vi "Teleop.vi"(10 "Match Info":T1={"Autonomous Elapsed Seconds"=0.0, "TeleOp Elapsed Seconds"=0.0, "Disabled Elapsed Seconds"=0.0, "Visited Autonomous"=FALSE, "Visited TeleOp"=FALSE, "Visited Disabled"=FALSE, "Autonomous Settings"={"Autonomous Style"=enum."Independent", "VI Refnum"=refnum}}, 11 "Call Context":T2) -> ()   [LabVIEW 2013]
doc: "This VI is called for each TeleOp packet received from the DS where the robot is not disabled. It is often used to read from the joysticks and update I/O or to update setpoints for timed control loops. It should complete and return within 20 milliseconds or it may miss DS packets."
uses:
  <vilib>/Rock Robotics/WPI/DriverStation/WPI_DriverStationDerivedRobotMode.ctl
  <vilib>/Rock Robotics/WPI/DriverStation/WPI_DriverStationMatch Info.ctl
  <vilib>/Rock Robotics/WPI/DriverStation/DriverStationLCD/WPI_DriverStationLCDLCDLine.ctl
  Robot Global Data.vi
  <vilib>/Rock Robotics/WPI/Joystick/WPI_JoystickGetSetRefNum.vi
  <vilib>/Rock Robotics/WPI/RobotDrive/WPI_RobotDriveGetSetRefNum.vi
  <vilib>/Rock Robotics/WPI/Solenoid/WPI_SolenoidSetEnum.vi
  <vilib>/Rock Robotics/WPI/Solenoid/WPI_SolenoidValue.ctl
panel:
  out "Numeric 1":dbl(slide) scale=0.0..100.0
  out "Boolean 2":bool
  out "Boolean 1":bool
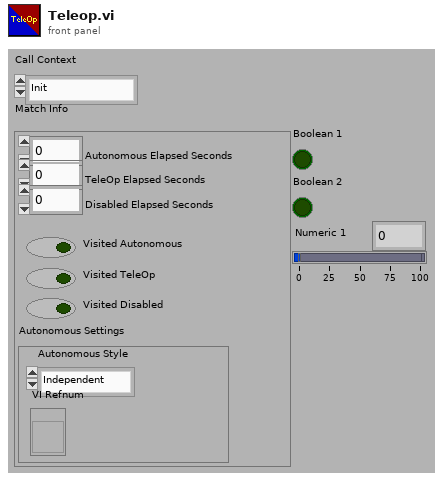
[diagram p1: front panel]
types:
  T1 = typedef "WPI_DriverStationMatch Info.ctl" = cluster{"Autonomous Elapsed Seconds":dbl, "TeleOp Elapsed Seconds":dbl, "Disabled Elapsed Seconds":dbl, "Visited Autonomous":bool, "Visited TeleOp":bool, "Visited Disabled":bool, "Autonomous Settings":cluster{"Autonomous Style":enum16{"Iterative", "Independent"}, "VI Refnum":refnum<vi>}}
  T2 = typedef "WPI_DriverStationDerivedRobotMode.ctl" = enum16{"Init", "Execute", "Stop"}
  T3 = typedef "WPI_DriverStationLCDLCDLine.ctl" = enum16{"Main - Line 1", "User - Line 2", "User - Line 3", "User - Line 4", "User - Line 5", "User - Line 6"}
  T4 = typedef "WPI_JoystickDevRef.ctl" = cluster{"Device":T5}
  T5 = typedef "WPI_JoystickDeviceEnum.ctl" = enum16{"USB 1", "USB 2", "USB 3", "USB 4", "Kinect 1", "Kinect 2"}
  T6 = typedef "WPI_JoystickButtonState.ctl" = cluster{"Button 1":bool, "Button 2":bool, "Button 3":bool, "Button 4":bool, "Button 5":bool, "Button 6":bool, "Button 7":bool, "Button 8":bool, "Button 9":bool, "Button 10":bool, "Button 11":bool, "Button 12":bool}
  T7 = cluster{"axis 1 (x)":dbl, "axis 2 (y)":dbl, "axis 3 (throttle)":dbl, "axis 4":dbl, "axis 5":dbl, "axis 6":dbl}
  T8 = typedef "WPI_SolenoidValue.ctl" = enum16{"Off", "On", "Forward", "Reverse"}
  T9 = typedef "WPI_SolenoidDevRef.ctl" = cluster{"DevStatus":errorcluster, "Solenoid Module":T10, "Forward Solenoid Channel":T11, "Reverse Solenoid Channel":T11}
  T10 = typedef "FPGA_TypedefSolenoidModule.ctl" = enum16{"Solenoid Module 1", "Solenoid Module 2"}
  T11 = typedef "WPI_SolenoidChannel.ctl" = enum8{"Solenoid 1", "Solenoid 2", "Solenoid 3", "Solenoid 4", "Solenoid 5", "Solenoid 6", "Solenoid 7", "Solenoid 8", "Invalid"}
  T12 = typedef "WPI_RobotDriveDevRef.ctl" = cluster{"DevStatus":errorcluster, "Motors[]":T13[], "Square Inputs":bool, "Max Output":dbl, "Isochronous":bool}
  T13 = typedef "WPI_MotorControlDeviceRef.ctl" = cluster{"DeviceStatus":errorcluster, "Type":enum16{"PWM", "CAN"}, "PWM":cluster{"Digital Module":T14, "PWM Channel":T15, "DeadBand":T16}, "CAN":cluster{"Device Number":u8, "Control Mode":T17, "Semaphore":T18, "Max Vout":dbl}, "Invert":bool, "TransformRef":T19, "InvTransformRef":T19}
  T14 = typedef "FPGA_TypedefDigitalModule.ctl" = enum16{"Digital Module 1", "Digital Module 2"}
  T15 = typedef "FPGA_DIOPWMChannel.ctl" = enum8{"PWM 1", "PWM 2", "PWM 3", "PWM 4", "PWM 5", "PWM 6", "PWM 7", "PWM 8", "PWM 9", "PWM 10", "Invalid"}
  T16 = typedef "WPI_PWMDeadband.ctl" = cluster{"Name":string, "maxPositivePwm":i32, "minPositivePwm":i32, "centerPwm":i32, "maxNegativePwm":i32, "minNegativePwm":i32, "angularRange":u16}
  T17 = typedef "WPI_CANJaguar_ControlMode.ctl" = enum8{"Percent VBus", "Current", "Speed", "Position", "Voltage"}
  T18 = typedef "Semaphore RefNum" = refnum<k1>
  T19 = typedef "WPI_PWMTransform_ConPane.ctl" = refnum<vi>
  T20 = enum16{"Reset", "Start", "Reset 2", "Manual", "Get ready to Fire", "Disengage Gearbox", "Ready to Fire", "Firing", "Firing Completed", "Reengage Gearbox"}
  T21 = typedef "WPI_DigitalInputDevRef.ctl" = cluster{"DevStatus":errorcluster, "DIO Channel":T22, "Digital Module":T14}
  T22 = typedef "FPGA_DIOChannel.ctl" = enum8{"DIO 1", "DIO 2", "DIO 3", "DIO 4", "DIO 5", "DIO 6", "DIO 7", "DIO 8", "DIO 9", "DIO 10", "DIO 11", "DIO 12", "DIO 13", "DIO 14", "Invalid"}
  T23 = typedef "WPI_ServoDeviceRef.ctl" = cluster{"DeviceStatus":errorcluster, "Digital Module":T14, "PWM Channel":T15, "DeadBand":T16}
  T24 = typedef "WPI_AnalogChannelDevRef.ctl" = cluster{"DevStatus":errorcluster, "Analog Module":T25, "Analog Channel":T26}
  T25 = typedef "FPGA_TypedefAnalogModule.ctl" = enum16{"Analog Module 1", "Analog Module 2"}
  T26 = typedef "FPGA_AIChannel.ctl" = enum8{"AI 1", "AI 2", "AI 3", "AI 4", "AI 5", "AI 6", "AI 7", "AI 8", "Invalid"}
  T27 = typedef "WPI_RelayDevRef.ctl" = cluster{"DevStatus":errorcluster, "Relay Channel":T28, "Digital Module":T14, "Relay Direction":T29}
  T28 = typedef "FPGA_DIORelayChannel.ctl" = enum8{"Relay 1", "Relay 2", "Relay 3", "Relay 4", "Relay 5", "Relay 6", "Relay 7", "Relay 8", "Invalid"}
  T29 = typedef "WPI_RelayDirection.ctl" = enum16{"Both directions", "Forward only", "Reverse only"}
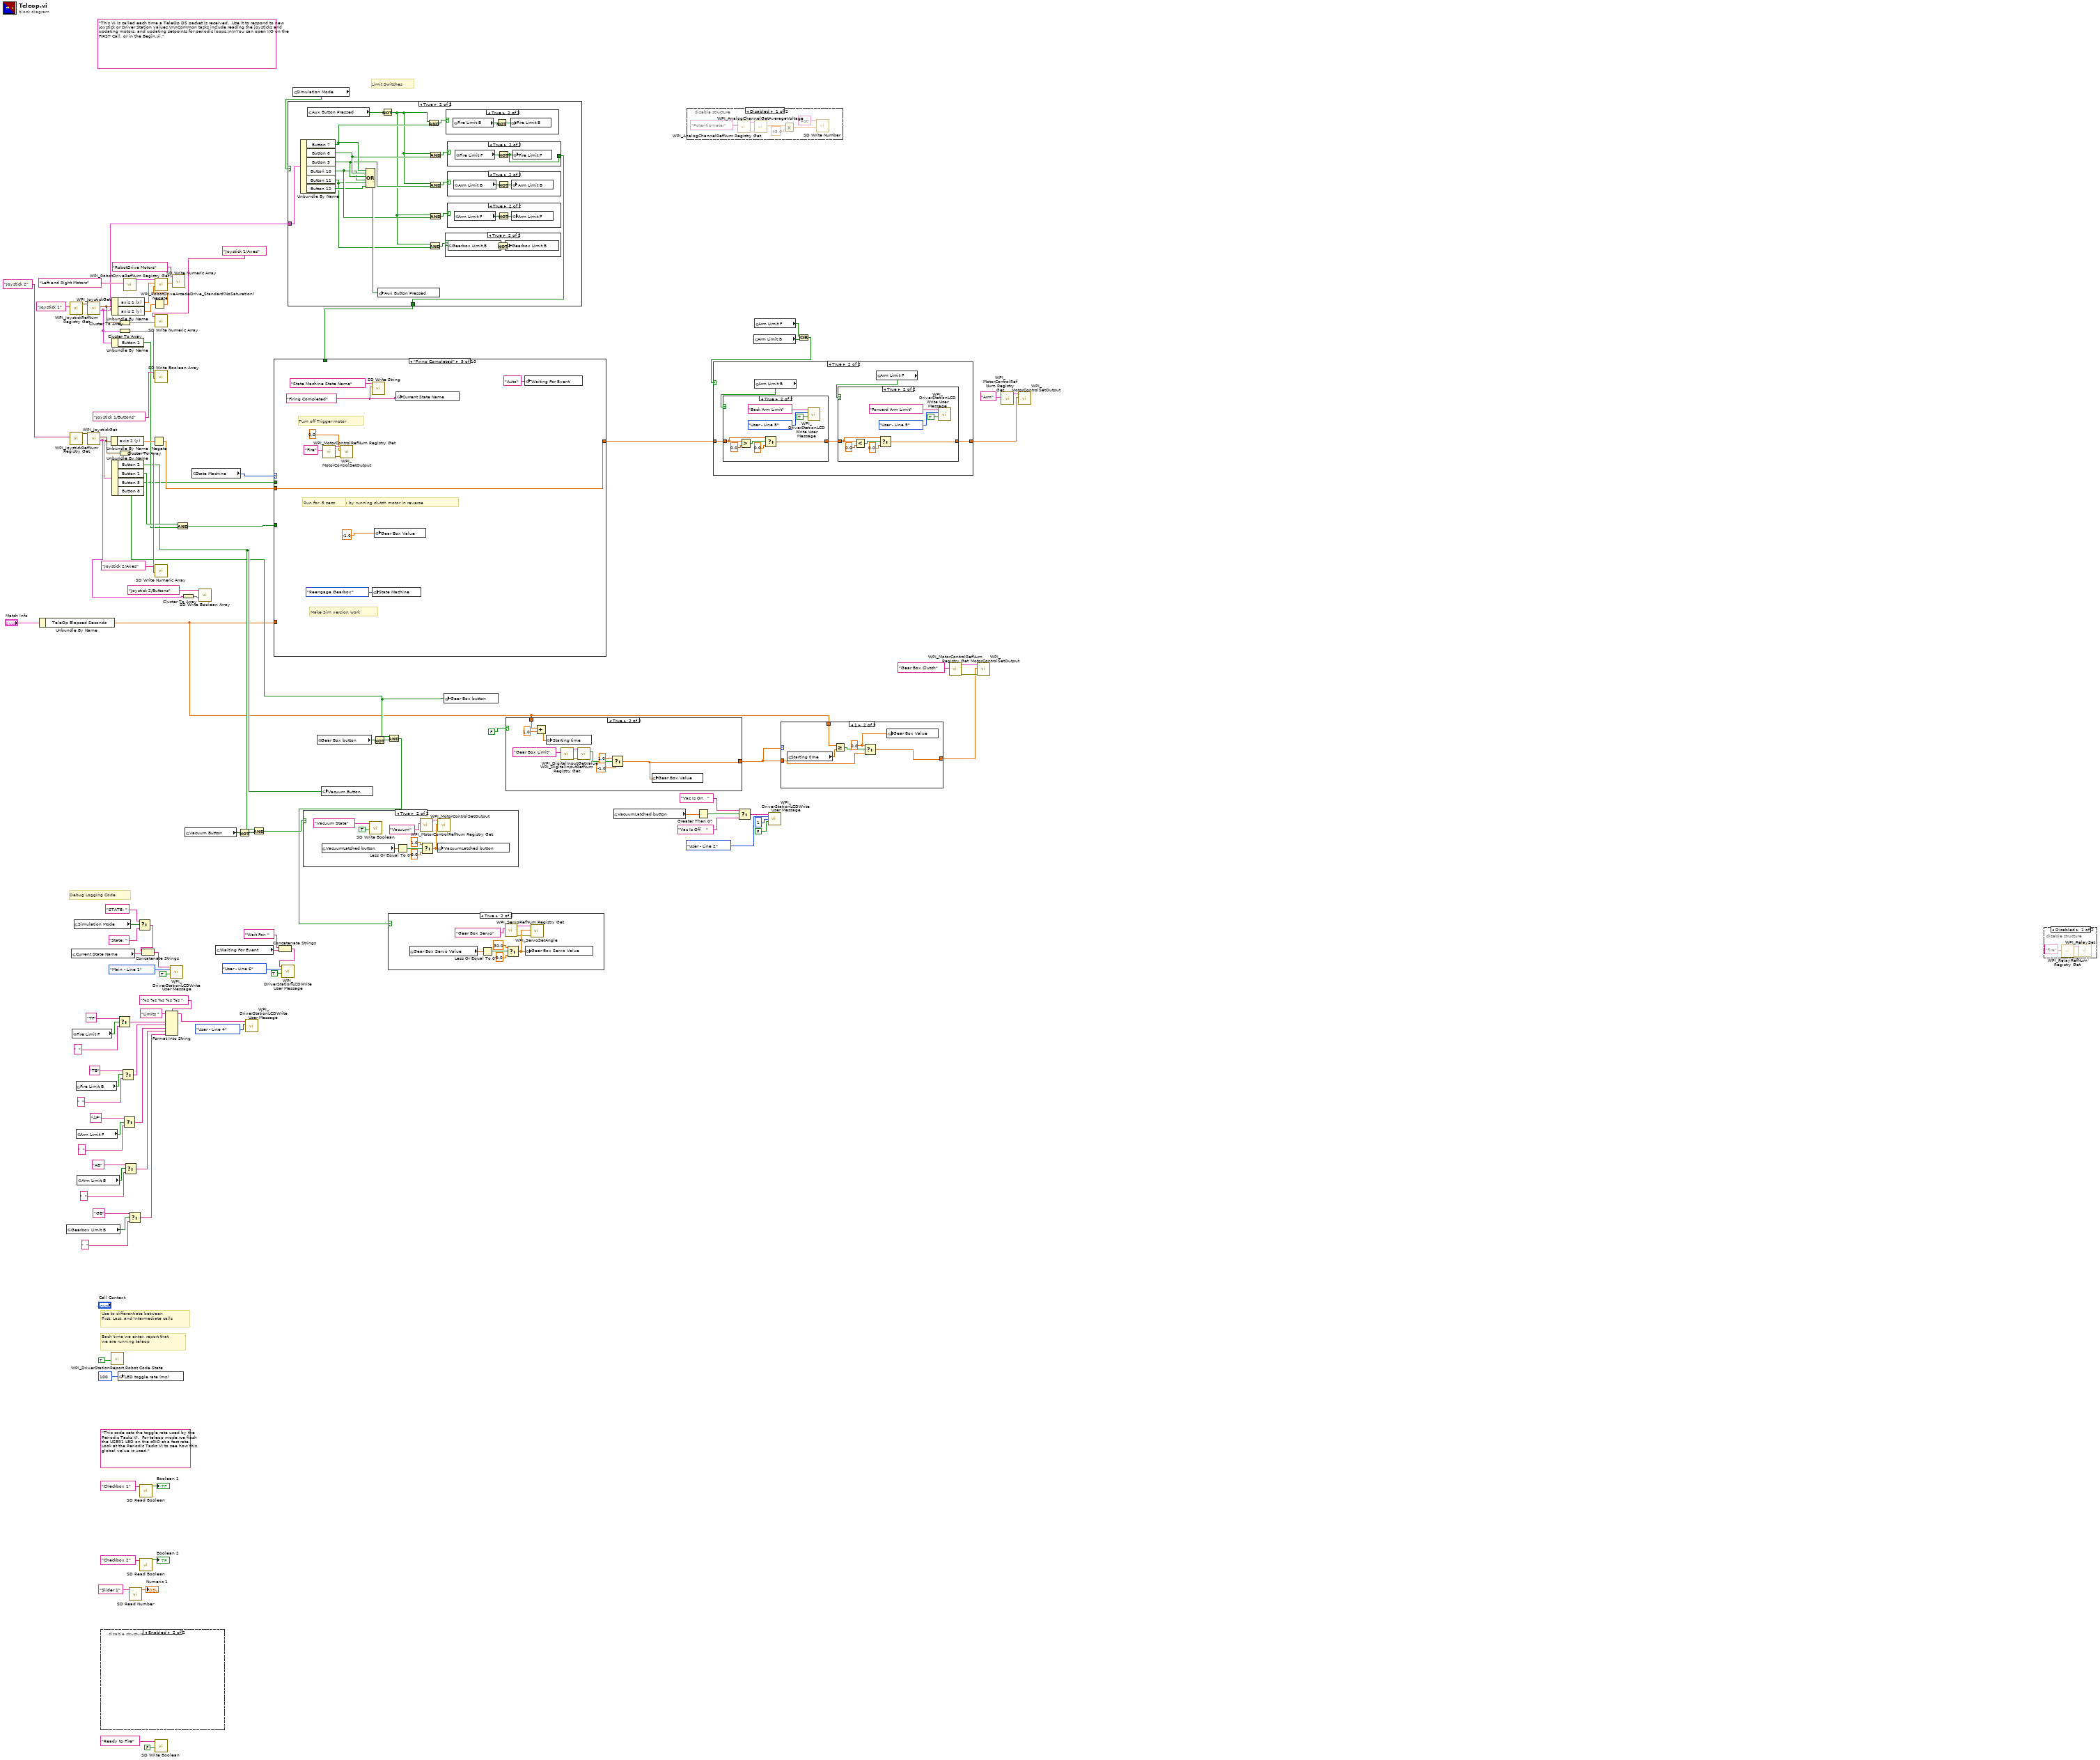
[diagram p0: block diagram]
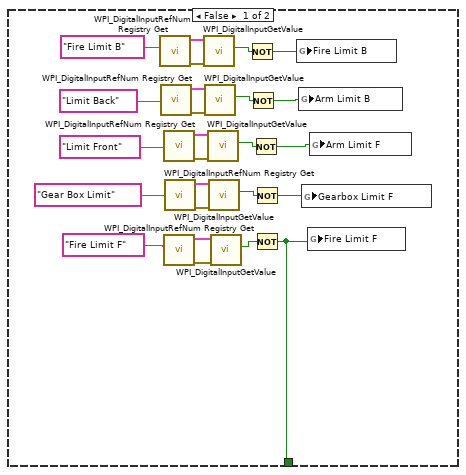
[diagram p3: hidden frame]
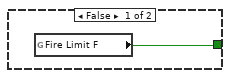
[diagram p7: hidden frame]
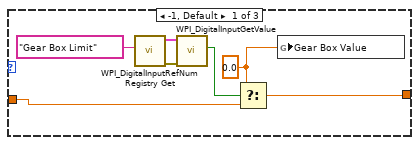
[diagram p9: hidden frame]
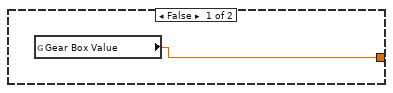
[diagram p11: hidden frame]
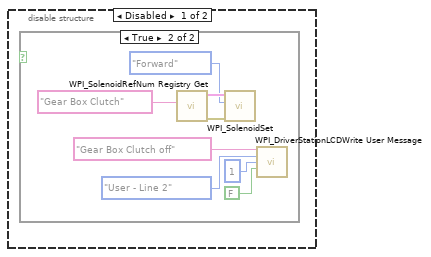
[diagram p18: hidden frame]
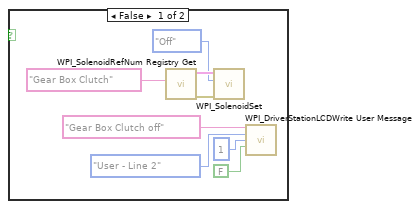
[diagram p19: hidden frame]
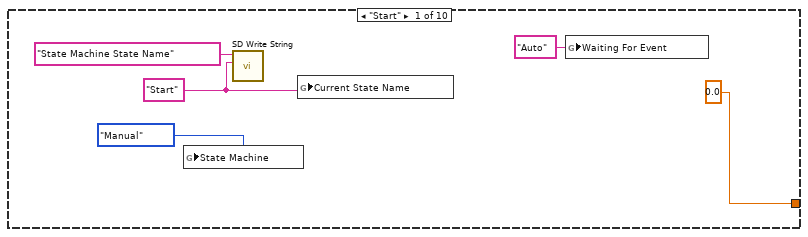
[diagram p20: hidden frame]
diagram:
  (unwired) "This code sets the toggle rate used by the Periodic Tasks VI.  For teleop mode we flash the USER1 LED on the cRIO at a fast rate.  Look at the Periodic Tasks VI to see how this global value is used."
  (unwired) "This VI is called each time a TeleOp DS packet is received.  Use it to respond to new joystick or Driver Station values.\n\nCommon tasks include reading the joysticks and updating motors, and updating setpoints for periodic loops.\n\nYou can open I/O on the FIRST Call, or in the Begin.vi."
  # "Limit Switches"
  # "Debug Logging Code"
  # "Each time we enter, report that\nwe are running teleop"
  # "Use to differentiate between\nFirst, Last, and Intermediate calls"
  n1 = Unbundle By Name("Match Info") -> ("TeleOp Elapsed Seconds"=w38:dbl)
  n2 = global read "Robot Global Data.vi" "Gearbox Limit B"() -> (w19:bool)
  n3 = call <vilib>:"WPI_JoystickRefNum Registry Get.vi"("refnum name"="Joystick 1") -> ("JoystickDevRef"=w105:T4)  [unwired: 1 in, 9 out]
  n4 = call <vilib>:"WPI_JoystickRefNum Registry Get.vi"("refnum name"="Joystick 2") -> ("JoystickDevRef"=w88:T4)  [unwired: 1 in, 9 out]
  n5 = global read "Robot Global Data.vi" "Current State Name"() -> (w53:string)
  n6 = global read "Robot Global Data.vi" "Fire Limit F"() -> (w23:bool)
  n7 = global read "Robot Global Data.vi" "Simulation Mode"() -> (w12:bool)
  n8 = global read "Robot Global Data.vi" "Fire Limit B"() -> (w22:bool)
  n9 = global read "Robot Global Data.vi" "Arm Limit F"() -> (w21:bool)
  n10 = global read "Robot Global Data.vi" "Arm Limit B"() -> (w20:bool)
  n11 = call <vilib>:"WPI_JoystickGet.vi"("JoystickDevRef"=w105) -> ("Buttons"=w8:T6, "Axes"=w100:T7)  [unwired: 1 in, 4 out]
  n12 = call <vilib>:"WPI_JoystickGet.vi"("JoystickDevRef"=w88) -> ("Buttons"=w82:T6, "Axes"=w85:T7)  [unwired: 1 in, 4 out]
  n13 = disable-structure shown="Enabled" {
    frame Disabled {
      n14 = case shown="True" {
        selector: _ -> [_ _]
        frame False {
          n15 = call <vilib>:"WPI_SolenoidRefNum Registry Get.vi"("refnum name"="Gear Box Clutch") -> ("error out"=w116:errorcluster, "SolenoidDevRef"=w117:T9)  [unwired: 9 in]
          n16 = call-poly <vilib>:"WPI_SolenoidSet.vi"("error in (no error)"=w116, "Value"=WPI_SolenoidValue."Off", "SolenoidDevRef"=w117) -> ()  [unwired: 7 in, 2 out]
          n17 = call <vilib>:"WPI_DriverStationLCDWrite User Message.vi"("line text"="Gear Box Clutch off", "line"=WPI_DriverStationLCDLCDLine."User - Line 2", "starting column"=i8 1, "clear line before write (T)"=FALSE) -> ()  [unwired: 11 in, 1 out]
        }
        frame True {
          n18 = call <vilib>:"WPI_SolenoidRefNum Registry Get.vi"("refnum name"="Gear Box Clutch") -> ("error out"=w124:errorcluster, "SolenoidDevRef"=w125:T9)  [unwired: 9 in]
          n19 = call-poly <vilib>:"WPI_SolenoidSet.vi"("error in (no error)"=w124, "Value"=WPI_SolenoidValue."Forward", "SolenoidDevRef"=w125) -> ()  [unwired: 7 in, 2 out]
          n20 = call <vilib>:"WPI_DriverStationLCDWrite User Message.vi"("line text"="Gear Box Clutch off", "line"=WPI_DriverStationLCDLCDLine."User - Line 2", "starting column"=i8 1, "clear line before write (T)"=FALSE) -> ()  [unwired: 11 in, 1 out]
        }
      }
    }
    frame Enabled {
    }
  }
  n21 = Unbundle By Name(w85) -> ("axis 2 (y)"=w81:dbl)
  n22 = call <vilib>:"WPI_DriverStationReport Robot Code State.vi"("TeleOp"=TRUE ("Autonomous")) -> ()  [unwired: 10 in, 1 out]
  n23 = Unbundle By Name(w100) -> ("axis 1 (x)"=w107:dbl, "axis 2 (y)"=w48:dbl)
  n24 = Unbundle By Name(w8) -> ("Button 1"=w79:bool)
  n25 = Unbundle By Name(w82) -> ("Button 2"=w70:bool, "Button 1"=w80:bool, "Button 5"=w56:bool, "Button 8"=w41:bool)
  n26 = Select(t="TF", s=w23, f="  ") -> (s? t:f=w29:string)
  n27 = global write "Robot Global Data.vi" "LED toggle rate (ms)"(u32 100 ("LED ms toggle rate")) -> ()
  n28 = Cluster To Array(cluster=w100) -> (array=w99:dbl[])
  n29 = Cluster To Array(cluster=w8) -> (array=w102:bool[])
  n30 = Cluster To Array(cluster=w85) -> (array=w84:dbl[])
  n31 = Select(t="TB", s=w22, f="  ") -> (s? t:f=w28:string)
  n32 = Select(t="AF", s=w21, f="  ") -> (s? t:f=w27:string)
  n33 = call <vilib>:"WPI_RobotDriveRefNum Registry Get.vi"("refnum name"="Left and Right Motors") -> ("RobotDriveDevRef"=w108:T12)  [unwired: 1 in, 9 out]
  n34 = Select(t="AB", s=w20, f="  ") -> (s? t:f=w26:string)
  n35 = Select(t="GB", s=w19, f="  ") -> (s? t:f=w25:string)
  n36 = call <vilib>:"SD Read Number.vi"("Name"="Slider 1" ("refnum name")) -> ("Numeric"=→"Numeric 1":dbl)  [unwired: 8 in, 2 out]
  n37 = Select(t="STATE: " ("line text"), s=w12, f="State: " ("line text")) -> (s? t:f=w9:string)
  n38 = call <vilib>:"SD Read Boolean.vi"("Name"="Checkbox 1" ("refnum name")) -> ("Boolean"=→"Boolean 1":bool)  [unwired: 8 in, 2 out]
  n39 = call <vilib>:"SD Read Boolean.vi"("Name"="Checkbox 2" ("refnum name")) -> ("Boolean"=→"Boolean 2":bool)  [unwired: 8 in, 2 out]
  n40 = Concatenate Strings(w9, w53) -> (w52:string)
  n41 = Negate(x=w81) -> (-x=w73:dbl)
  n42 = Negate(x=w48) -> (-x=w47:dbl)
  n43 = call <vilib>:"SD Write Boolean.vi"("Boolean"=FALSE, "Name"="Ready to Fire") -> ()  [unwired: 8 in, 2 out]
  n44 = call <vilib>:"WPI_RobotDriveArcadeDrive_Standard(NoSaturation).vi"("Y axis value"=w47, "X axis value"=w107, "RobotDriveDevRef"=w108) -> ("Motor Values"=w96:dbl[])  [unwired: 1 in, 7 out]
  n45 = call <vilib>:"SD Write Numeric Array.vi"("Numeric Array"=w99, "Name"="Joystick 1/Axes") -> ()  [unwired: 8 in, 2 out]
  n46 = call <vilib>:"SD Write Boolean Array.vi"("Boolean Array"=w102, "Name"="Joystick 1/Buttons") -> ()  [unwired: 8 in, 2 out]
  n47 = call <vilib>:"SD Write Numeric Array.vi"("Numeric Array"=w84, "Name"="Joystick 2/Axes") -> ()  [unwired: 8 in, 2 out]
  n48 = Format Into String(format string="%s %s %s %s %s " ("initial string"), initial string="Limits ", w29, w28, w27, w26, w25) -> (resulting string=w24:string)  [unwired: 1 in, 1 out]
  n49 = call <vilib>:"WPI_DriverStationLCDWrite User Message.vi"("line text"=w52, "line"=WPI_DriverStationLCDLCDLine."Main - Line 1", "clear line before write (T)"=TRUE) -> ()  [unwired: 12 in, 1 out]
  n50 = call <vilib>:"SD Write Numeric Array.vi"("Numeric Array"=w96, "Name"="RobotDrive Motors") -> ()  [unwired: 8 in, 2 out]
  n51 = And(x=w80, y=w79) -> (x .and. y?=w68:bool)
  n52 = Cluster To Array(cluster=w82) -> (array=w87:bool[])
  n53 = global read "Robot Global Data.vi" "Vacuum Button"() -> (w71:bool)
  n54 = global read "Robot Global Data.vi" "State Machine"() -> (w69:T20)
  n55 = call <vilib>:"SD Write Boolean Array.vi"("Boolean Array"=w87, "Name"="Joystick 2/Buttons") -> ()  [unwired: 8 in, 2 out]
  n56 = global read "Robot Global Data.vi" "Waiting For Event"() -> (w5:string)
  n57 = Not(x=w71) -> (.not. x?=w72:bool)
  n58 = call <vilib>:"WPI_DriverStationLCDWrite User Message.vi"("line text"=w24, "line"=WPI_DriverStationLCDLCDLine."User - Line 4") -> ()  [unwired: 13 in, 1 out]
  n59 = And(x=w70, y=w72) -> (x .and. y?=w66:bool)
  n60 = Concatenate Strings("Wait For: " ("string"), w5) -> (w3:string)
  n61 = call <vilib>:"WPI_DriverStationLCDWrite User Message.vi"("line text"=w3, "line"=WPI_DriverStationLCDLCDLine."User - Line 6", "clear line before write (T)"=TRUE) -> ()  [unwired: 12 in, 1 out]
  n62 = global read "Robot Global Data.vi" "Simulation Mode"() -> (w18:bool)
  n63 = case shown="True" w18 {
    tunnel: [w127 w152] -> w15
    tunnel: w8 -> [_ w167]
    frame False {
      n64 = call <vilib>:"WPI_DigitalInputRefNum Registry Get.vi"("refnum name"="Fire Limit B") -> ("error out"=w147:errorcluster, "DigitalInputDevRef"=w146:T21)  [unwired: 9 in]
      n65 = call <vilib>:"WPI_DigitalInputRefNum Registry Get.vi"("refnum name"="Limit Back") -> ("error out"=w143:errorcluster, "DigitalInputDevRef"=w142:T21)  [unwired: 9 in]
      n66 = call <vilib>:"WPI_DigitalInputRefNum Registry Get.vi"("refnum name"="Limit Front") -> ("error out"=w140:errorcluster, "DigitalInputDevRef"=w139:T21)  [unwired: 9 in]
      n67 = call <vilib>:"WPI_DigitalInputRefNum Registry Get.vi"("refnum name"="Fire Limit F") -> ("error out"=w150:errorcluster, "DigitalInputDevRef"=w151:T21)  [unwired: 9 in]
      n68 = call <vilib>:"WPI_DigitalInputRefNum Registry Get.vi"("refnum name"="Gear Box Limit") -> ("error out"=w136:errorcluster, "DigitalInputDevRef"=w135:T21)  [unwired: 9 in]
      n69 = call <vilib>:"WPI_DigitalInputGetValue.vi"("error in (no error)"=w147, "DigitalInputDevRef"=w146) -> ("Value"=w144:bool)  [unwired: 7 in, 2 out]
      n70 = call <vilib>:"WPI_DigitalInputGetValue.vi"("error in (no error)"=w143, "DigitalInputDevRef"=w142) -> ("Value"=w129:bool)  [unwired: 7 in, 2 out]
      n71 = call <vilib>:"WPI_DigitalInputGetValue.vi"("error in (no error)"=w140, "DigitalInputDevRef"=w139) -> ("Value"=w138:bool)  [unwired: 7 in, 2 out]
      n72 = call <vilib>:"WPI_DigitalInputGetValue.vi"("error in (no error)"=w136, "DigitalInputDevRef"=w135) -> ("Value"=w134:bool)  [unwired: 7 in, 2 out]
      n73 = call <vilib>:"WPI_DigitalInputGetValue.vi"("error in (no error)"=w150, "DigitalInputDevRef"=w151) -> ("Value"=w148:bool)  [unwired: 7 in, 2 out]
      n74 = Not(x=w144) -> (.not. x?=w128:bool)
      n75 = Not(x=w129) -> (.not. x?=w132:bool)
      n76 = Not(x=w138) -> (.not. x?=w131:bool)
      n77 = Not(x=w134) -> (.not. x?=w130:bool)
      n78 = Not(x=w148) -> (.not. x?=w127:bool)
      n79 = global write "Robot Global Data.vi" "Fire Limit B"(w128) -> ()
      n80 = global write "Robot Global Data.vi" "Arm Limit B"(w132) -> ()
      n81 = global write "Robot Global Data.vi" "Gearbox Limit F"(w130) -> ()
      n82 = global write "Robot Global Data.vi" "Fire Limit F"(w127) -> ()
      n83 = global write "Robot Global Data.vi" "Arm Limit F"(w131) -> ()
    }
    frame True {
      n84 = Unbundle By Name(w167) -> ("Button 7"=w165:bool, "Button 8"=w158:bool, "Button 9"=w157:bool, "Button 10"=w155:bool, "Button 11"=w153:bool, "Button 12"=w154:bool)
      n85 = global read "Robot Global Data.vi" "Aux Button Pressed"() -> (w166:bool)
      n86 = Compound Arithmetic op=OR(w165, w158, w157, w155, w153, w154) -> (w164:bool)
      n87 = global write "Robot Global Data.vi" "Aux Button Pressed"(w164) -> ()
      n88 = Not(x=w166) -> (.not. x?=w156:bool)
      n89 = And(x=w156, y=w165) -> (x .and. y?=w163:bool)
      n90 = And(x=w156, y=w153) -> (x .and. y?=w159:bool)
      n91 = And(x=w156, y=w158) -> (x .and. y?=w162:bool)
      n92 = And(x=w156, y=w157) -> (x .and. y?=w161:bool)
      n93 = And(x=w156, y=w155) -> (x .and. y?=w160:bool)
      n94 = case shown="True" w159 {
        frame False {
        }
        frame True {
          n95 = global read "Robot Global Data.vi" "Gearbox Limit B"() -> (w169:bool)
          n96 = Not(x=w169) -> (.not. x?=w168:bool)
          n97 = global write "Robot Global Data.vi" "Gearbox Limit B"(w168) -> ()
        }
      }
      n98 = case shown="True" w163 {
        frame False {
        }
        frame True {
          n99 = global read "Robot Global Data.vi" "Fire Limit B"() -> (w178:bool)
          n100 = Not(x=w178) -> (.not. x?=w177:bool)
          n101 = global write "Robot Global Data.vi" "Fire Limit B"(w177) -> ()
        }
      }
      n102 = case shown="True" w162 {
        tunnel: [w174 w175] -> w152
        frame False {
          n103 = global read "Robot Global Data.vi" "Fire Limit F"() -> (w174:bool)
        }
        frame True {
          n104 = global read "Robot Global Data.vi" "Fire Limit F"() -> (w176:bool)
          n105 = Not(x=w176) -> (.not. x?=w175:bool)
          n106 = global write "Robot Global Data.vi" "Fire Limit F"(w175) -> ()
        }
      }
      n107 = case shown="True" w161 {
        frame False {
        }
        frame True {
          n108 = global read "Robot Global Data.vi" "Arm Limit B"() -> (w173:bool)
          n109 = Not(x=w173) -> (.not. x?=w172:bool)
          n110 = global write "Robot Global Data.vi" "Arm Limit B"(w172) -> ()
        }
      }
      n111 = case shown="True" w160 {
        frame False {
        }
        frame True {
          n112 = global read "Robot Global Data.vi" "Arm Limit F"() -> (w171:bool)
          n113 = Not(x=w171) -> (.not. x?=w170:bool)
          n114 = global write "Robot Global Data.vi" "Arm Limit F"(w170) -> ()
        }
      }
    }
  }
  n115 = case shown="\"Firing Completed\"" w69 {
    selector: w69 -> [_ _ w209 _ _ _ _ w276 _ _]
    tunnel: w73 -> [_ _ _ w220 _ w257 w268 w284 w294 w300]
    tunnel: [0.0 w191 0.0 w220 0.0 w257 w268 w284 w294 w300] -> w67
    tunnel: w68 -> [_ _ _ _ _ _ w264 _ _ _]
    tunnel: w38 -> [_ w188 w202 _ w237 w252 _ _ _ _]
    tunnel: w56 -> [_ _ _ w219 _ _ _ _ _ _]
    tunnel: w15 -> [_ _ _ _ _ _ _ _ _ _]
    frame "Start" {
      w181 = "Start" ("line text")
      n116 = global write "Robot Global Data.vi" "State Machine"(T20."Manual" ("State Machine")) -> ()
      n117 = call <vilib>:"SD Write String.vi"("Table Prefix"=w181, "Name"="State Machine State Name") -> ()  [unwired: 8 in, 2 out]
      n118 = global write "Robot Global Data.vi" "Current State Name"(w181) -> ()
      n119 = global write "Robot Global Data.vi" "Waiting For Event"("Auto" ("Waiting For Event")) -> ()
    }
    frame "Reset" {
      w189 = "Reset" ("line text")
      # "Pull Arm back until hit Back limit\nthen turn power off"
      n120 = global read "Robot Global Data.vi" "Arm Limit B"() -> (w184:bool)
      n121 = Add(x=w188, y=1.0) -> (x+y=w186:dbl)
      n122 = global write "Robot Global Data.vi" "Starting time"(w186) -> ()
      n123 = case shown="True" w184 {
        frame False {
        }
        frame True {
          n124 = global write "Robot Global Data.vi" "State Machine"(T20."Reset 2" ("s? t:f")) -> ()
        }
      }
      n125 = call <vilib>:"SD Write String.vi"("Table Prefix"=w189, "Name"="State Machine State Name") -> ()  [unwired: 8 in, 2 out]
      n126 = global write "Robot Global Data.vi" "Current State Name"(w189) -> ()
      n127 = global write "Robot Global Data.vi" "Waiting For Event"("AB Limit" ("Waiting For Event")) -> ()
      n128 = call <vilib>:"SD Write Boolean.vi"("Boolean"=FALSE, "Name"="Ready to Fire") -> ()  [unwired: 8 in, 2 out]
      n129 = Select(t=0.5, s=w184, f=-0.7) -> (s? t:f=w191:dbl)
    }
    frame "Reset 2" {
      w204 = "Reset 2" ("line text")
      # "Reverse Trigger Motor until hit Back limit"
      n130 = global read "Robot Global Data.vi" "Starting time"() -> (w201:dbl)
      n131 = global read "Robot Global Data.vi" "Fire Limit B"() -> (w197:bool)
      n132 = Greater Or Equal?(x=w202, y=w201) -> (x >= y?=w200:bool)
      n133 = call <vilib>:"SD Write String.vi"("Table Prefix"=w204, "Name"="State Machine State Name") -> ()  [unwired: 8 in, 2 out]
      n134 = Or(x=w197, y=w200) -> (x .or. y?=w199:bool)
      n135 = global write "Robot Global Data.vi" "Current State Name"(w204) -> ()
      n136 = Select(t=T20."Manual" ("s? t:f"), s=w199, f=w209) -> (s? t:f=w208:T20)
      n137 = Select(t=0.0, s=w199, f=0.3) -> (s? t:f=w206:dbl)
      n138 = global write "Robot Global Data.vi" "State Machine"(w208) -> ()
      n139 = call <vilib>:"WPI_MotorControlRefNum Registry Get.vi"("refnum name"="Fire") -> ("error out"=w214:errorcluster, "MotorControlDevRef"=w213:T13)  [unwired: 9 in]
      n140 = call <vilib>:"WPI_MotorControlSetOutput.vi"("error in (no error)"=w214, "Output"=w206, "MotorControlDevRef"=w213) -> ()  [unwired: 6 in, 3 out]
      n141 = global write "Robot Global Data.vi" "Waiting For Event"("FB Limit" ("Waiting For Event")) -> ()
      n142 = call <vilib>:"SD Write Boolean.vi"("Boolean"=FALSE, "Name"="Ready to Fire") -> ()  [unwired: 8 in, 2 out]
    }
    frame "Manual", Default {
      w221 = "Manual" ("line text")
      # "If hit rear Arm limit switch, get ready to fire, \nelse if Reset button hit, start reset"
      n143 = global read "Robot Global Data.vi" "Arm Limit B"() -> (w218:bool)
      n144 = Or(x=w218, y=w219) -> (x .or. y?=w222:bool)
      n145 = case shown="True" w222 {
        tunnel: w218 -> [_ w231]
        frame False {
        }
        frame True {
          n146 = Select(t="Reason: Limit Back hit" ("line text"), s=w231, f="Reason Button 5 pressed:" ("line text")) -> (s? t:f=w226:string)
          n147 = Select(t=T20."Get ready to Fire" ("State Machine"), s=w231, f=T20."Reset" ("State Machine")) -> (s? t:f=w233:T20)
          n148 = global write "Robot Global Data.vi" "State Machine"(w233) -> ()
          n149 = call <vilib>:"WPI_DriverStationLCDWrite User Message.vi"("line text"=w226, "line"=WPI_DriverStationLCDLCDLine."User - Line 3", "clear line before write (T)"=TRUE) -> ()  [unwired: 12 in, 1 out]
        }
      }
      n150 = call <vilib>:"SD Write Boolean.vi"("Boolean"=FALSE, "Name"="Ready to Fire") -> ()  [unwired: 8 in, 2 out]
      n151 = call <vilib>:"SD Write String.vi"("Table Prefix"=w221, "Name"="State Machine State Name") -> ()  [unwired: 8 in, 2 out]
      n152 = global write "Robot Global Data.vi" "Current State Name"(w221) -> ()
      n153 = global write "Robot Global Data.vi" "Waiting For Event"("AB Limit | Btn 5" ("Waiting For Event")) -> ()
    }
    frame "Get ready to Fire" {
      w240 = "Get ready to Fire" ("line text")
      w246 = 0.0 ("f")
      # "Wait until hit gearbox limit switch"
      # "Disengage Gearbox"
      # "Turn Off Arm Motor"
      # "Turn Off Vacuum"
      n154 = global write "Robot Global Data.vi" "VacuumLatched button"(w246) -> ()
      n155 = Add(x=0.5 ("Starting time"), y=w237) -> (x+y=w238:dbl)
      n156 = call <vilib>:"WPI_MotorControlRefNum Registry Get.vi"("refnum name"="Vacuum") -> ("MotorControlDevRef"=w247:T13)  [unwired: 9 in, 1 out]
      n157 = global write "Robot Global Data.vi" "Starting time"(w238) -> ()
      n158 = call <vilib>:"WPI_MotorControlSetOutput.vi"("Output"=w246, "MotorControlDevRef"=w247) -> ()  [unwired: 7 in, 3 out]
      n159 = call <vilib>:"WPI_MotorControlRefNum Registry Get.vi"("refnum name"="Gear Box Clutch") -> ("MotorControlDevRef"=w245:T13)  [unwired: 9 in, 1 out]
      n160 = call <vilib>:"SD Write Boolean.vi"("Boolean"=TRUE, "Name"="Vacuum State") -> ()  [unwired: 8 in, 2 out]
      n161 = call <vilib>:"SD Write String.vi"("Table Prefix"=w240, "Name"="State Machine State Name") -> ()  [unwired: 8 in, 2 out]
      n162 = call <vilib>:"WPI_MotorControlSetOutput.vi"("Output"=1.0 ("Numeric"), "MotorControlDevRef"=w245) -> ()  [unwired: 7 in, 3 out]
      n163 = global write "Robot Global Data.vi" "Current State Name"(w240) -> ()
      n164 = global write "Robot Global Data.vi" "State Machine"(T20."Disengage Gearbox" ("State Machine")) -> ()
      n165 = global write "Robot Global Data.vi" "Waiting For Event"("Auto" ("Waiting For Event")) -> ()
    }
    frame "Disengage Gearbox" {
      w255 = "Disengage Gearbox" ("line text")
      # "When time completed, return to Manual control"
      n166 = global read "Robot Global Data.vi" "Starting time"() -> (w254:dbl)
      n167 = Greater Or Equal?(x=w252, y=w254) -> (x >= y?=w253:bool)
      n168 = call <vilib>:"SD Write String.vi"("Table Prefix"=w255, "Name"="State Machine State Name") -> ()  [unwired: 8 in, 2 out]
      n169 = case shown="True" w253 {
        frame False {
        }
        frame True {
          n170 = call <vilib>:"WPI_MotorControlRefNum Registry Get.vi"("refnum name"="Gear Box Clutch") -> ("MotorControlDevRef"=w261:T13)  [unwired: 9 in, 1 out]
          n171 = global write "Robot Global Data.vi" "State Machine"(T20."Ready to Fire" ("State Machine")) -> ()
          n172 = call <vilib>:"WPI_MotorControlSetOutput.vi"("Output"=0.0 ("Numeric"), "MotorControlDevRef"=w261) -> ()  [unwired: 7 in, 3 out]
        }
      }
      n173 = global write "Robot Global Data.vi" "Current State Name"(w255) -> ()
      n174 = global write "Robot Global Data.vi" "Waiting For Event"("Timer" ("Waiting For Event")) -> ()
    }
    frame "Ready to Fire" {
      w263 = "Ready to fire" ("line text")
      # "If both trigger btns pressed, fire"
      n175 = call <vilib>:"SD Write Boolean.vi"("Boolean"=FALSE, "Name"="Ready to Fire") -> ()  [unwired: 8 in, 2 out]
      n176 = call <vilib>:"SD Write String.vi"("Table Prefix"=w263, "Name"="State Machine State Name") -> ()  [unwired: 8 in, 2 out]
      n177 = global write "Robot Global Data.vi" "Current State Name"(w263) -> ()
      n178 = case shown="True" w264 {
        frame False {
        }
        frame True {
          n179 = global write "Robot Global Data.vi" "State Machine"(T20."Firing" ("State Machine")) -> ()
        }
      }
      n180 = global write "Robot Global Data.vi" "Waiting For Event"("Both Btn1s" ("Waiting For Event")) -> ()
    }
    frame "Firing" {
      w274 = "Firing" ("line text")
      # "Run Trigger motor forward until hit forward limit"
      n181 = global read "Robot Global Data.vi" "Fire Limit F"() -> (w270:bool)
      n182 = call <vilib>:"SD Write String.vi"("Table Prefix"=w274, "Name"="State Machine State Name") -> ()  [unwired: 8 in, 2 out]
      n183 = Select(t=T20."Firing Completed" ("s? t:f"), s=w270, f=w276) -> (s? t:f=w275:T20)
      n184 = global write "Robot Global Data.vi" "Current State Name"(w274) -> ()
      n185 = global write "Robot Global Data.vi" "State Machine"(w275) -> ()
      n186 = Select(t=0.0, s=w270, f=-0.8) -> (s? t:f=w278:dbl)
      n187 = call <vilib>:"WPI_MotorControlRefNum Registry Get.vi"("refnum name"="Fire") -> ("error out"=w283:errorcluster, "MotorControlDevRef"=w282:T13)  [unwired: 9 in]
      n188 = call <vilib>:"WPI_MotorControlSetOutput.vi"("error in (no error)"=w283, "Output"=w278, "MotorControlDevRef"=w282) -> ()  [unwired: 6 in, 3 out]
      n189 = global write "Robot Global Data.vi" "Waiting For Event"("FF Limit" ("Waiting For Event")) -> ()
      n190 = global write "Robot Global Data.vi" "Waiting For Event"("FF Limit" ("Waiting For Event")) -> ()
    }
    frame "Firing Completed" {
      w287 = "Firing Completed" ("line text")
      # "Make Sim version work"
      # "Run for .5 secs"
      # "Re-engage Gearbox by running clutch motor in reverse"
      # "Turn off Trigger motor"
      n191 = call <vilib>:"WPI_MotorControlRefNum Registry Get.vi"("refnum name"="Fire") -> ("error out"=w293:errorcluster, "MotorControlDevRef"=w292:T13)  [unwired: 9 in]
      n192 = call <vilib>:"WPI_MotorControlSetOutput.vi"("error in (no error)"=w293, "Output"=0.0, "MotorControlDevRef"=w292) -> ()  [unwired: 6 in, 3 out]
      n193 = call <vilib>:"SD Write String.vi"("Table Prefix"=w287, "Name"="State Machine State Name") -> ()  [unwired: 8 in, 2 out]
      n194 = global write "Robot Global Data.vi" "State Machine"(T20."Reengage Gearbox" ("State Machine")) -> ()
      n195 = global write "Robot Global Data.vi" "Gear Box Value"(-1.0 ("Numeric")) -> ()
      n196 = global write "Robot Global Data.vi" "Current State Name"(w287) -> ()
      n197 = global write "Robot Global Data.vi" "Waiting For Event"("Auto" ("Waiting For Event")) -> ()
    }
    frame "Reengage Gearbox" {
      w298 = "Reengage Gearbox" ("line text")
      # "Keep moving gearbox motor until hit limit switch"
      n198 = global read "Robot Global Data.vi" "Gearbox Limit B"() -> (w295:bool)
      n199 = global write "Robot Global Data.vi" "Waiting For Event"("GB Limit" ("Waiting For Event")) -> ()
      n200 = call <vilib>:"SD Write String.vi"("Table Prefix"=w298, "Name"="State Machine State Name") -> ()  [unwired: 8 in, 2 out]
      n201 = case shown="True" w295 {
        frame False {
        }
        frame True {
          n202 = global write "Robot Global Data.vi" "State Machine"(T20."Manual" ("State Machine")) -> ()
          n203 = call <vilib>:"WPI_MotorControlRefNum Registry Get.vi"("refnum name"="Gear Box Clutch") -> ("error out"=w301:errorcluster, "MotorControlDevRef"=w305:T13)  [unwired: 9 in]
          n204 = call <vilib>:"WPI_MotorControlSetOutput.vi"("error in (no error)"=w301, "Output"=0.0 ("Numeric"), "MotorControlDevRef"=w305) -> ()  [unwired: 6 in, 3 out]
        }
      }
      n205 = global write "Robot Global Data.vi" "Current State Name"(w298) -> ()
      n206 = global write "Robot Global Data.vi" "Waiting For Event"("GB Limit" ("Waiting For Event")) -> ()
    }
  }
  n207 = case shown="True" w66 {
    frame False {
    }
    frame True {
      n208 = global read "Robot Global Data.vi" "VacuumLatched button"() -> (w312:dbl)
      n209 = call <vilib>:"SD Write Boolean.vi"("Boolean"=TRUE, "Name"="Vacuum State") -> ()  [unwired: 8 in, 2 out]
      n210 = Less Or Equal To 0?(x=w312) -> (x <= 0?=w307:bool)
      n211 = call <vilib>:"WPI_MotorControlRefNum Registry Get.vi"("refnum name"="Vacuum") -> ("MotorControlDevRef"=w309:T13)  [unwired: 9 in, 1 out]
      n212 = Select(t=1.0 ("Numeric"), s=w307, f=0.0) -> (s? t:f=w308:dbl)
      n213 = call <vilib>:"WPI_MotorControlSetOutput.vi"("Output"=w308, "MotorControlDevRef"=w309) -> ()  [unwired: 7 in, 3 out]
      n214 = global write "Robot Global Data.vi" "VacuumLatched button"(w308) -> ()
    }
  }
  n215 = global read "Robot Global Data.vi" "Gear Box button"() -> (w42:bool)
  n216 = global write "Robot Global Data.vi" "Vacuum Button"(w70) -> ()
  n217 = Not(x=w42) -> (.not. x?=w43:bool)
  n218 = And(x=w41, y=w43) -> (x .and. y?=w2:bool)
  n219 = case shown="True" w2 {
    frame False {
    }
    frame True {
      n220 = global read "Robot Global Data.vi" "Gear Box Servo Value"() -> (w322:dbl)
      n221 = Less Or Equal To 0?(x=w322) -> (x <= 0?=w319:bool)
      n222 = call <vilib>:"WPI_ServoRefNum Registry Get.vi"("refnum name"="Gear Box Servo") -> ("error out"=w315:errorcluster, "ServoDeviceRef"=w316:T23)  [unwired: 9 in]
      n223 = Select(t=30.0 ("Numeric"), s=w319, f=0.0) -> (s? t:f=w317:dbl)
      n224 = global write "Robot Global Data.vi" "Gear Box Servo Value"(w317) -> ()
      n225 = call <vilib>:"WPI_ServoSetAngle.vi"("error in (no error)"=w315, "Angle"=w317, "ServoDeviceRef"=w316) -> ()  [unwired: 7 in, 2 out]
    }
  }
  n226 = global write "Robot Global Data.vi" "Gear Box button"(w41) -> ()
  n227 = case shown="True" FALSE {
    tunnel: w38 -> [_ w328]
    tunnel: [w323 w324] -> w39
    frame False {
      n228 = global read "Robot Global Data.vi" "Gear Box Value"() -> (w323:dbl)
    }
    frame True {
      n229 = Add(x=w328, y=1.0) -> (x+y=w332:dbl)
      n230 = global write "Robot Global Data.vi" "Starting time"(w332) -> ()
      n231 = call <vilib>:"WPI_DigitalInputRefNum Registry Get.vi"("refnum name"="Gear Box Limit") -> ("error out"=w330:errorcluster, "DigitalInputDevRef"=w331:T21)  [unwired: 9 in]
      n232 = call <vilib>:"WPI_DigitalInputGetValue.vi"("error in (no error)"=w330, "DigitalInputDevRef"=w331) -> ("Value"=w325:bool)  [unwired: 7 in, 2 out]
      n233 = Select(t=1.0, s=w325, f=-1.0) -> (s? t:f=w324:dbl)
      n234 = global write "Robot Global Data.vi" "Gear Box Value"(w324) -> ()
    }
  }
  n235 = global read "Robot Global Data.vi" "VacuumLatched button"() -> (w57:dbl)
  n236 = disable-structure shown="Disabled" {
    frame Disabled {
      n237 = call <vilib>:"WPI_AnalogChannelRefNum Registry Get.vi"("refnum name"="Potentiometer") -> ("error out"=w340:errorcluster, "AIDeviceRef"=w339:T24)  [unwired: 9 in]
      n238 = call <vilib>:"WPI_AnalogChannelGetAverageVoltage.vi"("error in (no error)"=w340, "AIDeviceRef"=w339) -> ("Voltage"=w335:dbl)  [unwired: 7 in, 2 out]
      n239 = Multiply(x=w335, y=45.0) -> (x*y=w334:dbl)
      n240 = call <vilib>:"SD Write Number.vi"("Numeric"=w334, "Name"="Pot") -> ()  [unwired: 8 in, 2 out]
    }
    frame Enabled {
    }
  }
  n241 = Greater Than 0?(x=w57) -> (x > 0?=w58:bool)
  n242 = Select(t="Vac Is On   ", s=w58, f="Vac Is Off    ") -> (s? t:f=w64:string)
  n243 = global read "Robot Global Data.vi" "Arm Limit B"() -> (w16:bool)
  n244 = global read "Robot Global Data.vi" "Arm Limit F"() -> (w17:bool)
  n245 = call <vilib>:"WPI_DriverStationLCDWrite User Message.vi"("line text"=w64, "line"=WPI_DriverStationLCDLCDLine."User - Line 2", "starting column"=i8 1, "clear line before write (T)"=FALSE) -> ()  [unwired: 11 in, 1 out]
  n246 = case shown="1" w39 {
    tunnel: [w343 w349 w354] -> w40
    tunnel: w39 -> [w342 w350 w354]
    tunnel: w38 -> [_ w353 _]
    frame -1, Default {
      w341 = 0.0 ("t")
      n247 = call <vilib>:"WPI_DigitalInputRefNum Registry Get.vi"("refnum name"="Gear Box Limit") -> ("error out"=w346:errorcluster, "DigitalInputDevRef"=w347:T21)  [unwired: 9 in]
      n248 = call <vilib>:"WPI_DigitalInputGetValue.vi"("error in (no error)"=w346, "DigitalInputDevRef"=w347) -> ("Value"=w344:bool)  [unwired: 7 in, 2 out]
      n249 = Select(t=w341, s=w344, f=w342) -> (s? t:f=w343:dbl)
      n250 = global write "Robot Global Data.vi" "Gear Box Value"(w341) -> ()
    }
    frame 1 {
      w348 = 0.0 ("t")
      n251 = global read "Robot Global Data.vi" "Starting time"() -> (w352:dbl)
      n252 = Greater Or Equal?(x=w353, y=w352) -> (x >= y?=w351:bool)
      n253 = Select(t=w348, s=w351, f=w350) -> (s? t:f=w349:dbl)
      n254 = global write "Robot Global Data.vi" "Gear Box Value"(w348) -> ()
    }
    frame 0 {
    }
  }
  n255 = Or(x=w17, y=w16) -> (x .or. y?=w74:bool)
  n256 = case shown="True" w74 {
    tunnel: w67 -> [w355 w360]
    tunnel: [w355 w358] -> w65
    frame False {
    }
    frame True {
      n257 = global read "Robot Global Data.vi" "Arm Limit B"() -> (w357:bool)
      n258 = case shown="True" w357 {
        tunnel: w360 -> [w370 w376]
        tunnel: [w370 w378] -> w359
        frame False {
        }
        frame True {
          n259 = Greater?(x=w376, y=0.0) -> (0:w374:bool)
          n260 = Select(t=w376, s=w374, f=0.0) -> (s? t:f=w378:dbl)
          n261 = call <vilib>:"WPI_DriverStationLCDWrite User Message.vi"("line text"="Back Arm Limit", "line"=WPI_DriverStationLCDLCDLine."User - Line 5", "clear line before write (T)"=TRUE) -> ()  [unwired: 12 in, 1 out]
        }
      }
      n262 = global read "Robot Global Data.vi" "Arm Limit F"() -> (w356:bool)
      n263 = case shown="True" w356 {
        tunnel: w359 -> [w361 w367]
        tunnel: [w361 w369] -> w358
        frame False {
        }
        frame True {
          n264 = Less?(x=w367, y=0.0) -> (x < y?=w365:bool)
          n265 = Select(t=w367, s=w365, f=0.0) -> (s? t:f=w369:dbl)
          n266 = call <vilib>:"WPI_DriverStationLCDWrite User Message.vi"("line text"="Forward Arm Limit", "line"=WPI_DriverStationLCDLCDLine."User - Line 5", "clear line before write (T)"=TRUE) -> ()  [unwired: 12 in, 1 out]
        }
      }
    }
  }
  n267 = call <vilib>:"WPI_MotorControlRefNum Registry Get.vi"("refnum name"="Gear Box Clutch") -> ("error out"=w46:errorcluster, "MotorControlDevRef"=w44:T13)  [unwired: 9 in]
  n268 = call <vilib>:"WPI_MotorControlSetOutput.vi"("error in (no error)"=w46, "Output"=w40, "MotorControlDevRef"=w44) -> ()  [unwired: 6 in, 3 out]
  n269 = call <vilib>:"WPI_MotorControlRefNum Registry Get.vi"("refnum name"="Arm") -> ("MotorControlDevRef"=w76:T13)  [unwired: 9 in, 1 out]
  n270 = call <vilib>:"WPI_MotorControlSetOutput.vi"("Output"=w65, "MotorControlDevRef"=w76) -> ()  [unwired: 7 in, 3 out]
  n271 = disable-structure shown="Disabled" {
    frame Disabled {
      n272 = call <vilib>:"WPI_RelayRefNum Registry Get.vi"("refnum name"="fire") -> ("error out"=w380:errorcluster, "RelayDevRef"=w381:T27)  [unwired: 9 in]
      n273 = call <vilib>:"WPI_RelaySet.vi"("error in (no error)"=w380, "RelayDevRef"=w381) -> ()  [unwired: 8 in, 2 out]
    }
    frame Enabled {
    }
  }
